vi "Update Values Array.vi"(7 "index of element":i32, 8 "error in (no error)":errorcluster, 10 "Assert Data":T1, 11 "Values in":variant[](array[variant])) -> (0 "error out":errorcluster, 3 "Values out":variant[](array[variant]))   [LabVIEW 2016, in "AssertEngine.lvlib" / "AssertEngine.lvclass"]
doc: "Updates the Values array, either by building a new object with new attributes, or by replacing an existing one at a known index."
uses:
  AssertEngine.lvclass
  Log Assert/Assert Data.ctl
  AssertEngine.lvlib
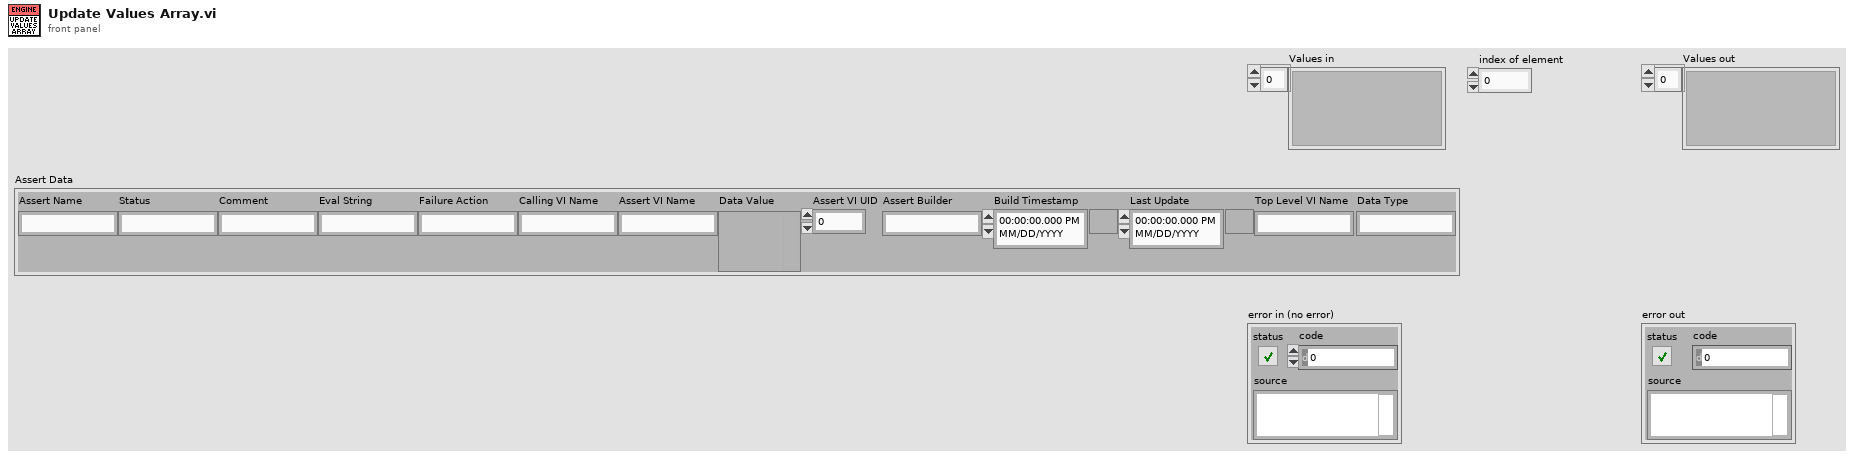
[diagram p1: front panel]
types:
  T1 = typedef "AssertEngine.lvlib/Assert Data.ctl" = cluster{"Assert Name":string, "Status":string, "Comment":string, "Eval String":string, "Failure Action":string, "Calling VI Name":string, "Assert VI Name":string, "Data Value":variant, "Assert VI UID":i32, "Assert Builder":string, "Build Timestamp":timestamp, "Last Update":timestamp, "Top Level VI Name":string, "Data Type":string}
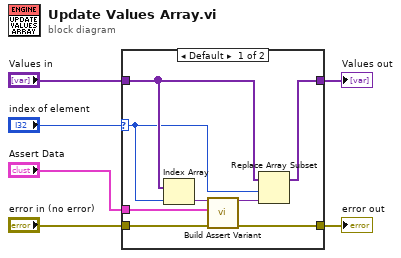
[diagram p0: block diagram]
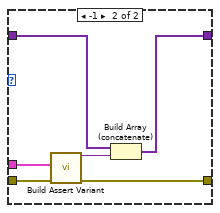
[diagram p2: hidden frame]
diagram:
  n1 = case shown="Default" "index of element" {
    selector: "index of element" -> [w9 _]
    tunnel: "Values in" -> [w11 w19]
    tunnel: "error in (no error)" -> [w13 w20]
    tunnel: [w12 w17] -> w3
    tunnel: [w8 w16] -> w4
    tunnel: "Assert Data" -> [w7 w15]
    frame Default {
      n2 = Index Array(array=w11, index=w9) -> (element=w14:variant)
      n3 = call "Build Assert Variant.vi"("error in (no error)"=w13, "Assert Data"=w7, "Assert Variant in"=w14) -> ("error out"=w12:errorcluster, "Assert Variant out"=w10:variant)  [unwired: 7 in]
      n4 = Replace Array Subset(array=w11, new element=w10, index=w9) -> (w8:variant[])
    }
    frame -1 {
      n5 = call "Build Assert Variant.vi"("error in (no error)"=w20, "Assert Data"=w15) -> ("error out"=w17:errorcluster, "Assert Variant out"=w18:variant)  [unwired: 8 in]
      n6 = Build Array (concatenate)(w19, w18) -> (w16:variant[])
    }
  }
  "Values out" <- w4
  "error out" <- w3
